vi "Initialize Attributes.vi"(8 "error in (no error)":errorcluster, 10 "Attribute Data":variant, 11 "CS++SeqEditor in":refnum<class "CS++SeqEditor.lvclass">) -> (0 "error out":errorcluster, 2 "Found?":bool, 3 "CS++SeqEditor out":refnum<class "CS++SeqEditor.lvclass">)   [LabVIEW 2016, in "CS++SeqEditor.lvlib" / "CS++SeqEditor.lvclass"]
doc: "Initialize object attribute.\n\nUnique resources should be allocated elsewhere!"
uses:
  CS++SeqEditor.lvclass
  CS++SeqEditor.lvclass/CS++SeqEditor.ctl
  CSPP_Core/Actors/CS++GUIActor/CS++GUIActor.lvclass
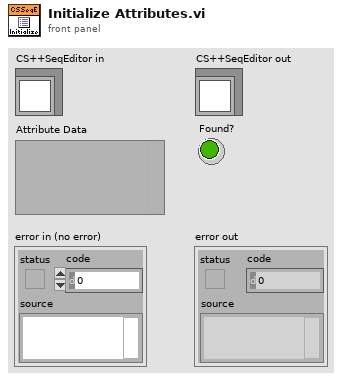
[diagram p1: front panel]
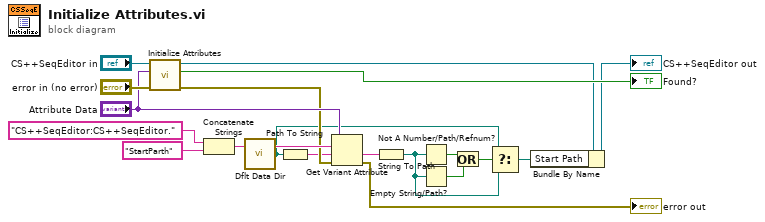
[diagram p0: block diagram]
diagram:
  n1 = call-parent "Initialize Attributes.vi"("error in (no error)"="error in (no error)", "Attribute Data"="Attribute Data", "CS++GUIActor in"="CS++SeqEditor in") -> ("error out"=w12:errorcluster, "Found?"=→"Found?":bool, "CS++GUIActor out"=w7:refnum<class "CS++SeqEditor.lvclass">)  [unwired: 6 in]
  n2 = Concatenate Strings("CS++SeqEditor:CS++SeqEditor.", "StartParth" ("string")) -> (w13:string)
  n3 = call <vilib>:"Dflt Data Dir.vi"() -> ("App:Default Data Directory"=w3:path)
  n4 = Path To String(path=w3) -> (string=w11:string)
  n5 = Get Variant Attribute(Variant="Attribute Data", name=w13, default value (empty Variant)=w11, error in=w12) -> (value=w10:string, error out=→"error out":errorcluster)  [unwired: 2 out]
  n6 = String To Path(string=w10) -> (path=w4:path)
  n7 = Not A Number/Path/Refnum?(number/path/refnum=w4) -> (NaN/Path/Refnum?=w9:bool)
  n8 = Empty String/Path?(string/path=w4) -> (empty?=w8:bool)
  n9 = Or(x=w9, y=w8) -> (x .or. y?=w5:bool)
  n10 = Select(t=w3, s=w5, f=w4) -> (s? t:f=w2:path)
  n11 = Bundle By Name(cluster=w7, "Start Path"=w2) -> (→"CS++SeqEditor out":refnum<class "CS++SeqEditor.lvclass">)
